vi "Configure Frequency Start Stop.vi"(8 "error in (no error)":errorcluster {"code" format="%.0x"}, 9 "stop frequency":dbl caption="stop frequency (Hz)", 10 "start frequency":dbl caption="start frequency (Hz)", 11 "instrument handle":refnum<k15>) -> (0 "error out":errorcluster {"code" format="%.0x"}, 3 "instrument handle out":refnum<k15>)   [LabVIEW 2009, in "Keysight XSAn.lvlib"]
doc: "This VI configures the frequency range of the IviSpecAn using start frequency and stop frequency. If start frequency is equal to the stop frequency, then the spectrum analyzer is in time-domain mode. In auto-coupled mode, resolution bandwidth (RBW), video bandwidth (VBW), and sweep time may be affected by this function.\n\nSupported Models: M9290A, N8973B, N8974B, N8975B, N8976B, N9000A, N9000B, N9010A, N9010B, N9020A, N9020B, N9030A, N9030B, N9038A, N9040B, N9041B, SPN9003A, SPN9026A"
uses:
  <instrlib>/Keysight XSAn/Keysight XSAn.lvlib
  AgXSAn.dll
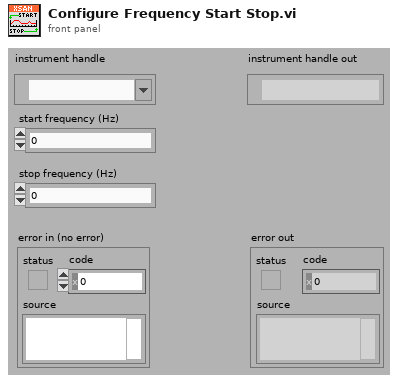
[diagram p1: front panel]
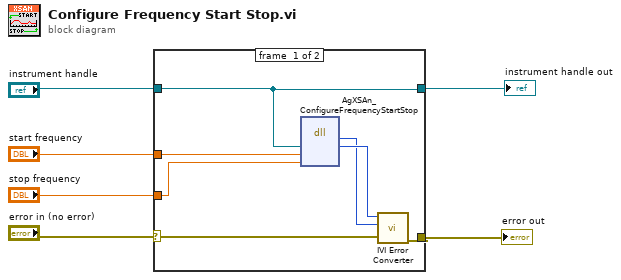
[diagram p0: block diagram]
diagram:
  n1 = case shown="No Error" "error in (no error)" {
    selector: "error in (no error)" -> [w9 w15]
    tunnel: [w12 w15] -> w5
    tunnel: "instrument handle" -> [w10 w14]
    tunnel: [w10 w14] -> w3
    tunnel: "start frequency" -> [w8 _]
    tunnel: "stop frequency" -> [w7 _]
    frame #0 {
      n2 = dll-call lib="AgXSAn**.dll" fn="AgXSAn_ConfigureFrequencyStartStop" ("LabVIEW:IviSpecAn_ConfigureFrequencyStartStop")("instrument handle"=w10, "start frequency"=w8, "stop frequency"=w7) -> ("Status"=w11:i32, "instrument handle"=w13:u32)  [unwired: 5 in, 2 out]
      n3 = call <instrlib>:"IVI Error Converter.vi"("error in (no error)"=w9, "IVI error code (0)"=w11, "instrument handle"=w13) -> ("error out"=w12:errorcluster)  [unwired: 7 in, 1 out]
    }
    frame #1 {
    }
  }
  "error out" <- w5
  "instrument handle out" <- w3
